vi "Enqueue Message.vi"   [LabVIEW 2020, in "MVA Message Mapper.lvlib"]
doc: "For a regular message, enqueue the message. For a priority message, enqueue it at the front of the queue."
uses:
  <vilib>/gpm_packages/@cs/Bus-message-mapper/Source/MVA Message Mapper.lvlib
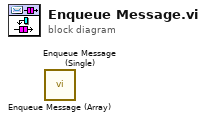
[diagram p0: block diagram]
diagram:
  n1 = call <vilib>:"Enqueue Message (Array).vi"() -> ()  [unwired: 10 in, 2 out]
  n2 = call <vilib>:"Enqueue Message (Single).vi"() -> ()  [unwired: 10 in, 2 out]
